vi "z_N[Psi_tau,tau_0,T,W,t_0]_Analytical.vi"(4 "Use z[0]":bool, 5 "tau_0":ext, 6 "t0":ext, 7 "Harmonic f":ext, 8 "N":i32, 9 "W":ext, 10 "T":ext, 11 "tau":ext) -> (3 "z_n,N,W(tau,tau_0)":cxt)   [LabVIEW 2021, in "Phasor.lvlib"]
uses:
  Phasor.lvlib
  Math/ix/ix (EXT).vi
  Math/Math.lvlib
  fbf690f7-72af-4727-ac41-3040469e0afe.vi
  4ade6035-4148-484c-a1e7-0dabd058c3dc.vi
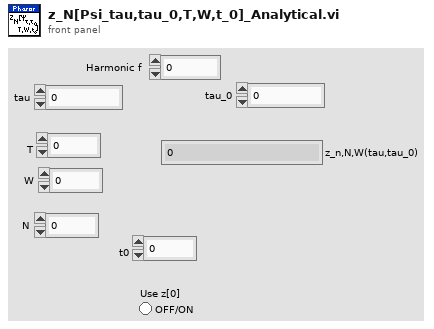
[diagram p1: front panel]
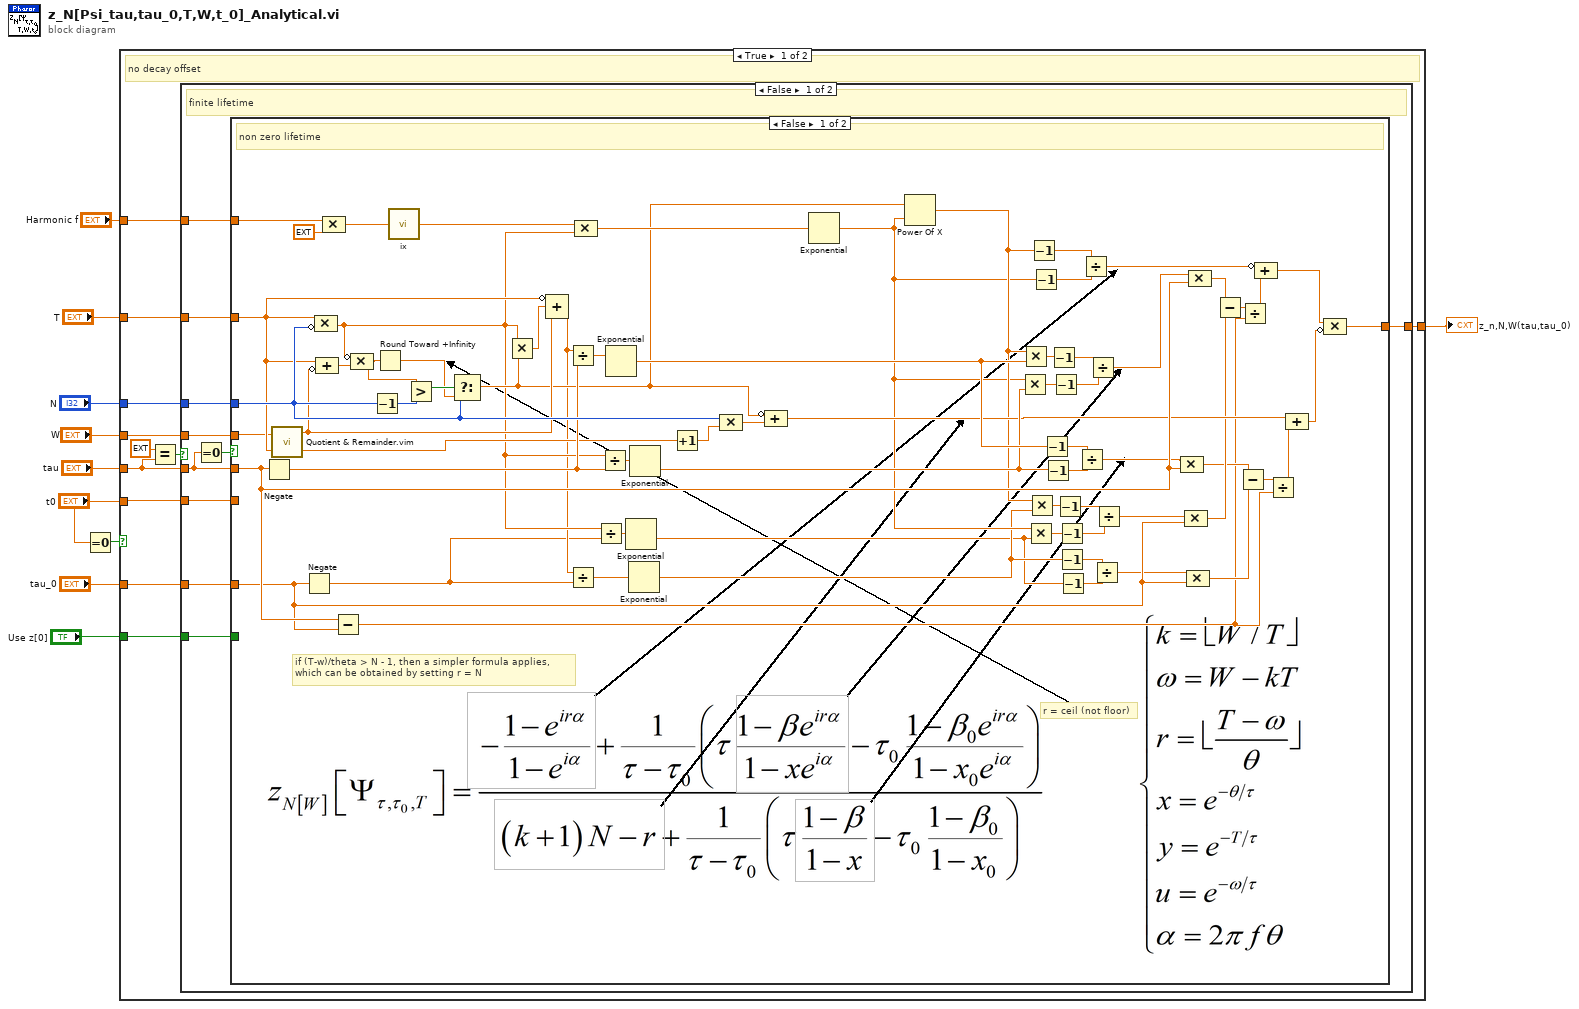
[diagram p0: block diagram]
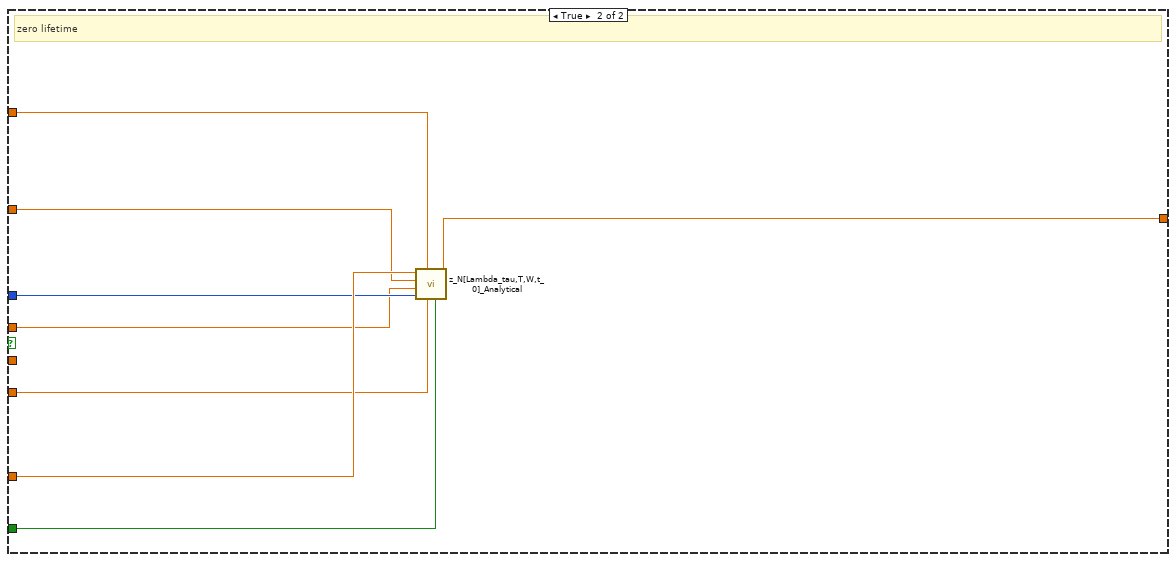
[diagram p2: hidden frame]
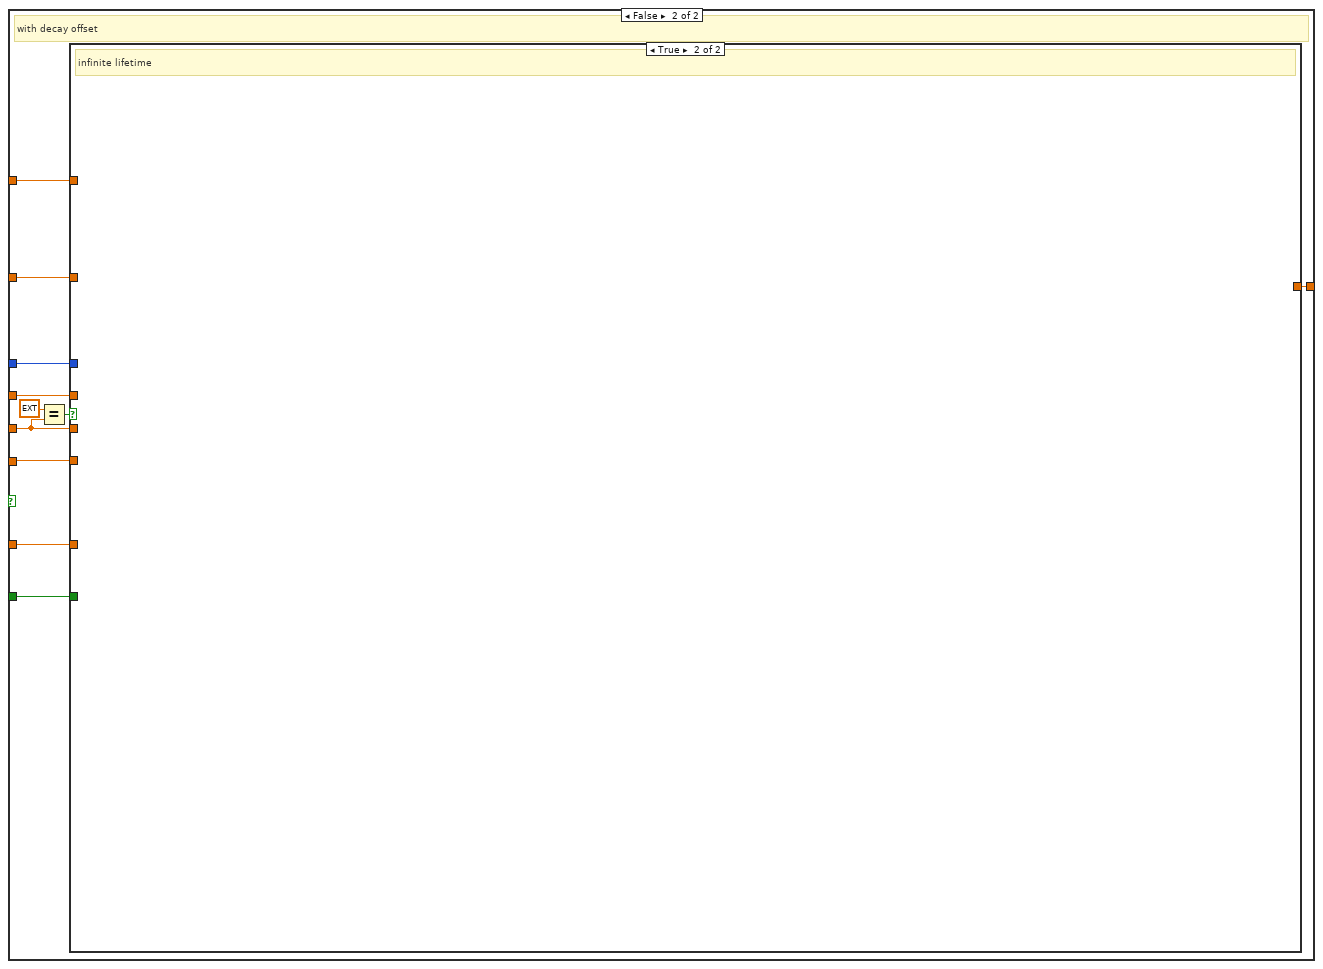
[diagram p4: hidden frame]
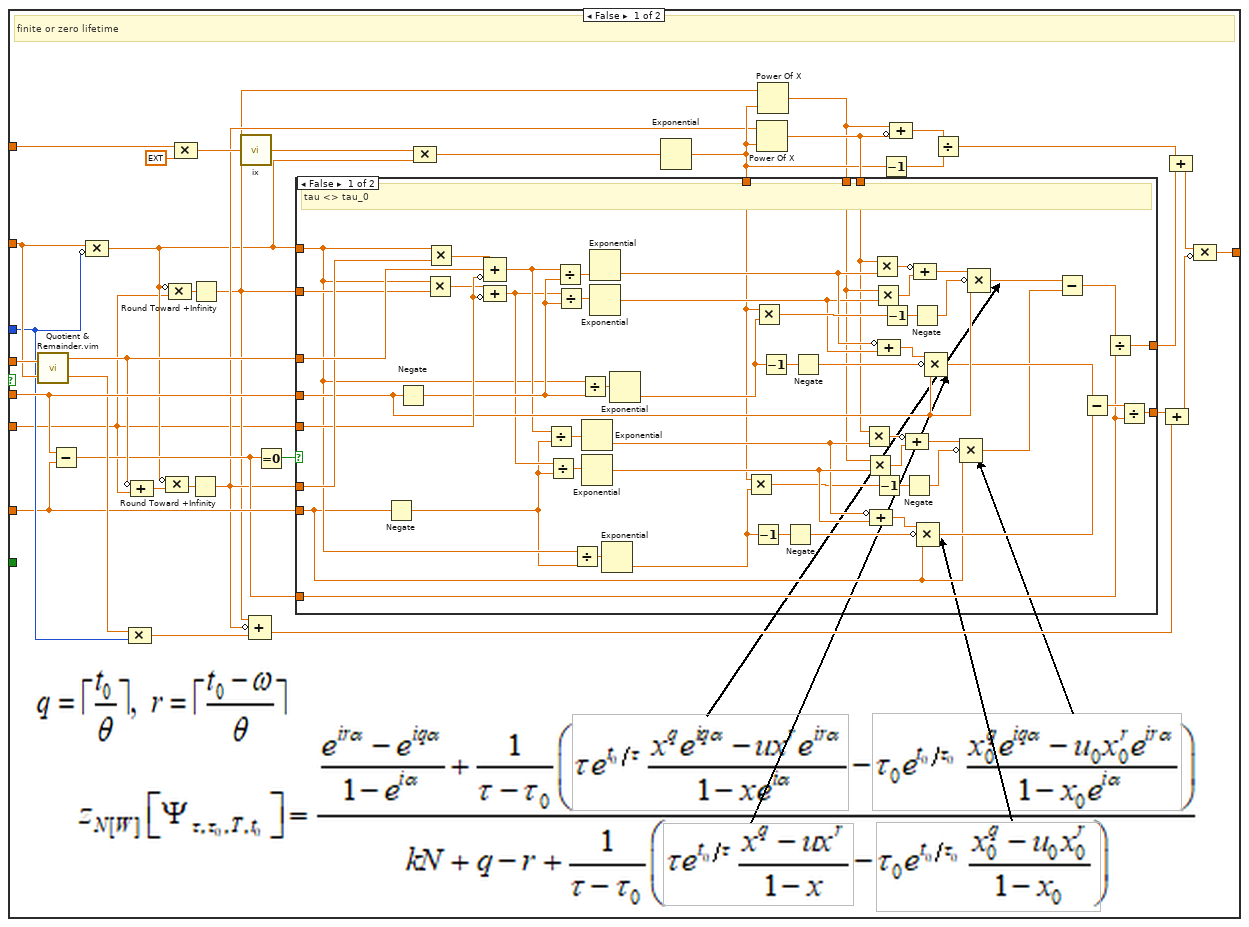
[diagram p5: hidden frame]
diagram:
  n1 = Equal To 0?(x="t0") -> (x = 0?=w3:bool)
  n2 = case shown="True" w3 {
    tunnel: "tau" -> [w16 w112]
    tunnel: "Harmonic f" -> [w21 w117]
    tunnel: [w20 w116] -> w8
    tunnel: "W" -> [w19 w115]
    tunnel: "T" -> [w17 w113]
    tunnel: "N" -> [w18 w114]
    tunnel: "t0" -> [w11 w107]
    tunnel: "Use z[0]" -> [w13 w109]
    tunnel: "tau_0" -> [w12 w108]
    frame True {
      # "no decay offset"
      n3 = Equal?(x=ext inf, y=w16) -> (x = y?=w14:bool)
      n4 = case shown="False" w14 {
        tunnel: w21 -> [w26 _]
        tunnel: [w31 _] -> w20
        tunnel: w19 -> [w30 _]
        tunnel: w18 -> [w29 _]
        tunnel: w17 -> [w28 _]
        tunnel: w16 -> [w27 _]
        tunnel: w13 -> [w24 _]
        tunnel: w12 -> [w23 _]
        tunnel: w11 -> [w22 _]
        frame False {
          # "finite lifetime"
          n5 = Equal To 0?(x=w27) -> (x = 0?=w25:bool)
          n6 = case shown="False" w25 {
            tunnel: [w98 w99] -> w31
            tunnel: w30 -> [w32 w102]
            tunnel: w29 -> [w97 w104]
            tunnel: w28 -> [w96 w103]
            tunnel: w27 -> [w95 _]
            tunnel: w26 -> [w94 w106]
            tunnel: w24 -> [_ w100]
            tunnel: w23 -> [w93 w105]
            tunnel: w22 -> [_ w101]
            frame False {
              # "r = ceil (not floor)"
              # "if (T-w)/theta > N - 1, then a simpler formula applies,\nwhich can be obtained by setting r = N"
              # "non zero lifetime"
              n7 = Negate(x=w95) -> (-x=w79:ext)
              n8 = call "Quotient & Remainder.vim"("y"=w96, "x"=w32) -> ("E(x/y)"=w63:ext, "x - E(x/y)y"=w80:ext)
              n9 = Negate(x=w93) -> (-x=w45:ext)
              n10 = Compound Arithmetic op=MULTIPLY(w96, invert w97) -> (w59:ext)
              n11 = Compound Arithmetic op=ADD(w96, invert w80) -> (w81:ext)
              n12 = Compound Arithmetic op=MULTIPLY(w94, ext 6.283185307179586477) -> (w34:ext)
              n13 = Subtract(x=w95, y=w93) -> (x-y=w36:ext)
              n14 = Compound Arithmetic op=MULTIPLY(invert w59, w81) -> (w73:ext)
              n15 = Decrement(x=w97) -> (x-1=w77:i32)
              n16 = Round Toward +Infinity(x=w73) -> (ceil(x): smallest int >= x=w75:ext)
              n17 = call-poly "ix.vi"("x (1)"=w34) -> ("i.(x)"=w33:cxt)
              n18 = Greater?(x=w73, y=w77) -> (0:w76:bool)
              n19 = Select(t=w97, s=w76, f=w75) -> (s? t:f=w74:ext)
              n20 = Multiply(x=w59, y=w74) -> (x*y=w66:ext)
              n21 = Compound Arithmetic op=ADD(invert w96, w66, w80) -> (w58:ext)
              n22 = Divide(x=w58, y=w79) -> (x/y=w65:ext)
              n23 = Divide(x=w58, y=w45) -> (x/y=w57:ext)
              n24 = Compound Arithmetic op=MULTIPLY(w33, w59) -> (w82:cxt)
              n25 = Divide(x=w59, y=w45) -> (x/y=w60:ext)
              n26 = Divide(x=w59, y=w79) -> (x/y=w64:ext)
              n27 = Exponential(1:w65) -> (0:w90:ext)
              n28 = Exponential(1:w60) -> (0:w41:ext)
              n29 = Exponential(1:w57) -> (0:w42:ext)
              n30 = Exponential(1:w64) -> (0:w87:ext)
              n31 = Increment(x=w63) -> (x+1=w61:ext)
              n32 = Compound Arithmetic op=MULTIPLY(w97, w61) -> (w62:ext)
              n33 = Compound Arithmetic op=ADD(invert w74, w62) -> (w86:ext)
              n34 = Exponential(1:w82) -> (0:w49:cxt)
              n35 = Power Of X(1:w49, 2:w74) -> (0:w50:cxt)
              n36 = Multiply(x=w49, y=w87) -> (x*y=w70:cxt)
              n37 = Multiply(x=w50, y=w90) -> (x*y=w69:cxt)
              n38 = Multiply(x=w49, y=w41) -> (x*y=w54:cxt)
              n39 = Multiply(x=w50, y=w42) -> (x*y=w53:cxt)
              n40 = Decrement(x=w50) -> (x-1=w78:cxt)
              n41 = Decrement(x=w49) -> (x-1=w85:cxt)
              n42 = Decrement(x=w90) -> (x-1=w68:ext)
              n43 = Decrement(x=w87) -> (x-1=w67:ext)
              n44 = Decrement(x=w69) -> (x-1=w72:cxt)
              n45 = Decrement(x=w70) -> (x-1=w71:cxt)
              n46 = Decrement(x=w53) -> (x-1=w56:cxt)
              n47 = Decrement(x=w54) -> (x-1=w55:cxt)
              n48 = Decrement(x=w42) -> (x-1=w51:ext)
              n49 = Decrement(x=w41) -> (x-1=w52:ext)
              n50 = Divide(x=w68, y=w67) -> (x/y=w89:ext)
              n51 = Divide(x=w78, y=w85) -> (x/y=w84:cxt)
              n52 = Divide(x=w72, y=w71) -> (x/y=w92:cxt)
              n53 = Divide(x=w51, y=w52) -> (x/y=w40:ext)
              n54 = Divide(x=w56, y=w55) -> (x/y=w48:cxt)
              n55 = Compound Arithmetic op=MULTIPLY(w89, w95) -> (w39:ext)
              n56 = Compound Arithmetic op=MULTIPLY(w48, w93) -> (w46:cxt)
              n57 = Compound Arithmetic op=MULTIPLY(w40, w93) -> (w38:ext)
              n58 = Compound Arithmetic op=MULTIPLY(w92, w95) -> (w47:cxt)
              n59 = Subtract(x=w47, y=w46) -> (x-y=w44:cxt)
              n60 = Subtract(x=w39, y=w38) -> (x-y=w37:ext)
              n61 = Divide(x=w44, y=w36) -> (x/y=w43:cxt)
              n62 = Compound Arithmetic op=ADD(invert w84, w43) -> (w91:cxt)
              n63 = Divide(x=w37, y=w36) -> (x/y=w35:ext)
              n64 = Compound Arithmetic op=ADD(w86, w35) -> (w83:ext)
              n65 = Compound Arithmetic op=MULTIPLY(w91, invert w83) -> (w98:cxt)
            }
            frame True {
              # "zero lifetime"
              n66 = call "z_N[Lambda_tau,T,W,t_0]_Analytical.vi"("Use z[0]"=w100, "t0"=w101, "Harmonic f"=w106, "N"=w104, "W"=w102, "T"=w103, "tau"=w105) -> ("z_n,N,W(tau)"=w99:cxt)  [unwired: 4 in]
            }
          }
        }
        frame True {
          # "infinite lifetime"
        }
      }
    }
    frame False {
      # "with decay offset"
      n67 = Equal?(x=ext inf, y=w112) -> (x = y?=w110:bool)
      n68 = case shown="True" w110 {
        tunnel: w117 -> [w148 _]
        tunnel: [w151 _] -> w116
        tunnel: w115 -> [w150 _]
        tunnel: w114 -> [w133 _]
        tunnel: w113 -> [w149 _]
        tunnel: w112 -> [w134 _]
        tunnel: w109 -> [_ _]
        tunnel: w108 -> [w130 _]
        tunnel: w107 -> [w118 _]
        frame False {
          # "finite or zero lifetime"
          n69 = call "Quotient & Remainder.vim"("y"=w149, "x"=w150) -> ("E(x/y)"=w132:ext, "x - E(x/y)y"=w129:ext)
          n70 = Subtract(x=w134, y=w130) -> (x-y=w123:ext)
          n71 = Compound Arithmetic op=MULTIPLY(w149, invert w133) -> (w119:ext)
          n72 = Compound Arithmetic op=MULTIPLY(w132, w133) -> (w126:ext)
          n73 = Compound Arithmetic op=ADD(invert w129, w118) -> (w127:ext)
          n74 = Compound Arithmetic op=MULTIPLY(invert w119, w127) -> (w128:ext)
          n75 = Compound Arithmetic op=MULTIPLY(invert w119, w118) -> (w131:ext)
          n76 = Compound Arithmetic op=MULTIPLY(w148, ext 6.283185307179586477) -> (w139:ext)
          n77 = Round Toward +Infinity(x=w128) -> (ceil(x): smallest int >= x=w122:ext)
          n78 = Round Toward +Infinity(x=w131) -> (ceil(x): smallest int >= x=w121:ext)
          n79 = call-poly "ix.vi"("x (1)"=w139) -> ("i.(x)"=w138:cxt)
          n80 = Compound Arithmetic op=ADD(w121, invert w122, w126) -> (w124:ext)
          n81 = Equal To 0?(x=w123) -> (x = 0?=w125:bool)
          n82 = Compound Arithmetic op=MULTIPLY(w138, w119) -> (w142:cxt)
          n83 = Exponential(1:w142) -> (0:w136:cxt)
          n84 = Power Of X(1:w136, 2:w122) -> (0:w137:cxt)
          n85 = Power Of X(1:w136, 2:w121) -> (0:w120:cxt)
          n86 = case shown="False" w125 {
            tunnel: [w202 _] -> w141
            tunnel: [w200 _] -> w140
            tunnel: w137 -> [w155 _]
            tunnel: w136 -> [w157 _]
            tunnel: w134 -> [w181 _]
            tunnel: w119 -> [w159 _]
            tunnel: w130 -> [w152 _]
            tunnel: w129 -> [w199 _]
            tunnel: w123 -> [w198 _]
            tunnel: w122 -> [w197 _]
            tunnel: w121 -> [w194 _]
            tunnel: w118 -> [w195 _]
            tunnel: w120 -> [w156 _]
            frame False {
              # "tau <> tau_0"
              n87 = Negate(x=w152) -> (-x=w158:ext)
              n88 = Negate(x=w181) -> (-x=w192:ext)
              n89 = Multiply(x=w159, y=w194) -> (x*y=w193:ext)
              n90 = Multiply(x=w159, y=w197) -> (x*y=w206:ext)
              n91 = Compound Arithmetic op=ADD(w206, w199, invert w195) -> (w161:ext)
              n92 = Compound Arithmetic op=ADD(w193, invert w195) -> (w160:ext)
              n93 = Divide(x=w161, y=w158) -> (x/y=w162:ext)
              n94 = Divide(x=w160, y=w158) -> (x/y=w165:ext)
              n95 = Divide(x=w161, y=w192) -> (x/y=w205:ext)
              n96 = Divide(x=w160, y=w192) -> (x/y=w191:ext)
              n97 = Divide(x=w159, y=w158) -> (x/y=w163:ext)
              n98 = Divide(x=w159, y=w192) -> (x/y=w204:ext)
              n99 = Exponential(1:w162) -> (0:w171:ext)
              n100 = Exponential(1:w165) -> (0:w172:ext)
              n101 = Exponential(1:w205) -> (0:w184:ext)
              n102 = Exponential(1:w191) -> (0:w183:ext)
              n103 = Exponential(1:w163) -> (0:w174:ext)
              n104 = Exponential(1:w204) -> (0:w180:ext)
              n105 = Multiply(x=w157, y=w174) -> (x*y=w168:cxt)
              n106 = Decrement(x=w174) -> (x-1=w175:ext)
              n107 = Multiply(x=w157, y=w180) -> (x*y=w188:cxt)
              n108 = Decrement(x=w180) -> (x-1=w179:ext)
              n109 = Negate(x=w175) -> (-x=w176:ext)
              n110 = Negate(x=w179) -> (-x=w178:ext)
              n111 = Multiply(x=w155, y=w171) -> (x*y=w164:cxt)
              n112 = Multiply(x=w156, y=w172) -> (x*y=w166:cxt)
              n113 = Compound Arithmetic op=ADD(invert w171, w172) -> (w173:ext)
              n114 = Multiply(x=w155, y=w184) -> (x*y=w196:cxt)
              n115 = Multiply(x=w156, y=w183) -> (x*y=w190:cxt)
              n116 = Decrement(x=w168) -> (x-1=w169:cxt)
              n117 = Compound Arithmetic op=ADD(invert w184, w183) -> (w182:ext)
              n118 = Decrement(x=w188) -> (x-1=w187:cxt)
              n119 = Negate(x=w169) -> (-x=w170:cxt)
              n120 = Compound Arithmetic op=ADD(invert w164, w166) -> (w167:cxt)
              n121 = Negate(x=w187) -> (-x=w186:cxt)
              n122 = Compound Arithmetic op=ADD(invert w196, w190) -> (w189:cxt)
              n123 = Compound Arithmetic op=MULTIPLY(w173, invert w176, w152) -> (w153:ext)
              n124 = Compound Arithmetic op=MULTIPLY(w182, invert w178, w181) -> (w177:ext)
              n125 = Compound Arithmetic op=MULTIPLY(w167, invert w170, w152) -> (w154:cxt)
              n126 = Compound Arithmetic op=MULTIPLY(w189, invert w186, w181) -> (w185:cxt)
              n127 = Subtract(x=w185, y=w154) -> (x-y=w203:cxt)
              n128 = Subtract(x=w177, y=w153) -> (x-y=w201:ext)
              n129 = Divide(x=w203, y=w198) -> (x/y=w202:cxt)
              n130 = Divide(x=w201, y=w198) -> (x/y=w200:ext)
            }
            frame True {
              # "tau = tau_0"
            }
          }
          n131 = Decrement(x=w136) -> (x-1=w145:cxt)
          n132 = Compound Arithmetic op=ADD(w120, invert w137) -> (w135:cxt)
          n133 = Divide(x=w135, y=w145) -> (x/y=w144:cxt)
          n134 = Compound Arithmetic op=ADD(w140, w124) -> (w143:ext)
          n135 = Compound Arithmetic op=ADD(w144, w141) -> (w147:cxt)
          n136 = Compound Arithmetic op=MULTIPLY(w147, invert w143) -> (w151:cxt)
        }
        frame True {
          # "infinite lifetime"
        }
      }
    }
  }
  "z_n,N,W(tau,tau_0)" <- w8
